vi "Set SplitterPosition.vi"(8 "error in (no error)":errorcluster caption="错误输入（无错误）", 10 "Position(relative)":dbl, 11 "PanelDataNode 输入":refnum<class "PanelDataNode.lvclass"> caption="DNL_LabVIEW Object in") -> (0 "error out":errorcluster caption="错误输出", 3 "PanelDataNode 输出":refnum<class "PanelDataNode.lvclass"> caption="DNL_LabVIEW Object out")   [LabVIEW 2016, in "PanelDataNode.lvclass"]
uses:
  PanelDataNode.lvclass
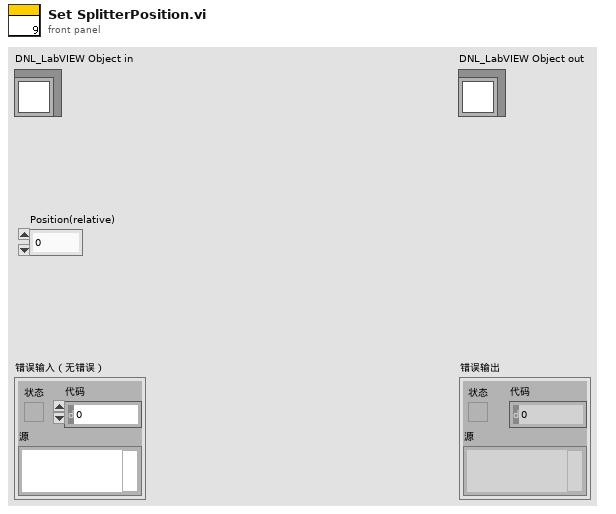
[diagram p1: front panel]
types:
  T1 = typedef "LVBoundsTypeDef.ctl" = cluster{"Width":u32, "Height":u32}
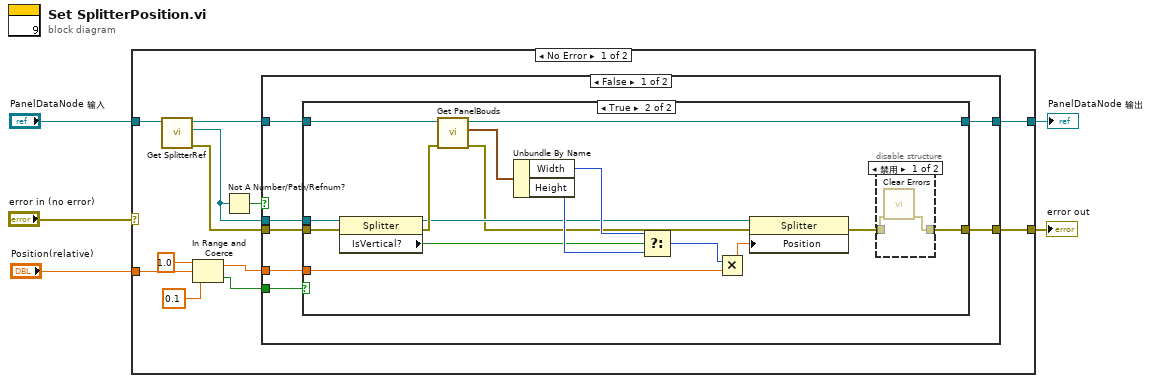
[diagram p0: block diagram]
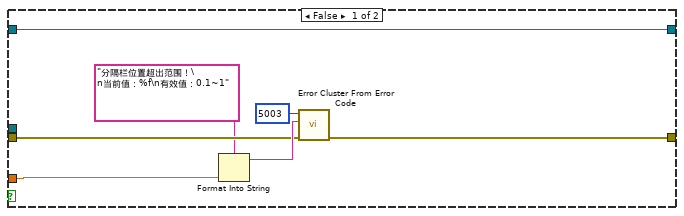
[diagram p2: hidden frame]
diagram:
  n1 = case shown="No Error" "error in (no error)" {
    selector: "error in (no error)" -> [_ w54]
    tunnel: [w13 w54] -> w4
    tunnel: [w14 w53] -> w2
    tunnel: "PanelDataNode 输入" -> [w17 w53]
    tunnel: "Position(relative)" -> [w8 _]
    frame No Error {
      n2 = call "Get SplitterRef.vi"("PanelDataNode 输入"=w17) -> ("error out"=w15:errorcluster, "Splitter"=w11:refnum<vi>, "PanelDataNode 输出"=w16:refnum<class "PanelDataNode.lvclass">)  [unwired: 8 in]
      n3 = In Range and Coerce(upper limit=1.0 ("上限"), x=w8, lower limit=0.1 ("下限")) -> (coerced(x)=w7:dbl, In Range?=w6:bool)
      n4 = Not A Number/Path/Refnum?(number/path/refnum=w11) -> (NaN/Path/Refnum?=w12:bool)
      n5 = case shown="False" w12 {
        tunnel: w16 -> [w24 w52]
        tunnel: w7 -> [w23 _]
        tunnel: w11 -> [w22 _]
        tunnel: w15 -> [w21 w51]
        tunnel: [w20 w52] -> w14
        tunnel: [w19 w51] -> w13
        tunnel: w6 -> [w18 _]
        frame False {
          n6 = case shown="True" w18 {
            tunnel: w24 -> [w25 w47]
            tunnel: w23 -> [w30 w42]
            tunnel: w22 -> [_ w41]
            tunnel: w21 -> [w29 w40]
            tunnel: [w25 w38] -> w20
            tunnel: [w28 w32] -> w19
            frame False {
              n7 = Format Into String(format string="分隔栏位置超出范围！\n当前值：%f\n有效值：0.1~1" ("格式字符串"), w30) -> (resulting string=w31:string)  [unwired: 2 in, 1 out]
              n8 = call <vilib>:"Error Cluster From Error Code.vi"("error in (no error)"=w29, "error message (\"\")"=w31, "error code (0)"=5003) -> ("error out"=w28:errorcluster)  [unwired: 6 in]
            }
            frame True {
              n9 = property class="Splitter"(reference=w41, error in=w40) -> (reference out=w36:refnum<vi>, error out=w39:errorcluster, "IsVertical?"=w37:bool)
              n10 = call "Get PanelBouds.vi"("error in (no error)"=w39, "PanelDataNode 输入"=w47) -> ("error out"=w35:errorcluster, "Bounds"=w44:T1, "PanelDataNode 输出"=w38:refnum<class "PanelDataNode.lvclass">)  [unwired: 7 in]
              n11 = Unbundle By Name(w44) -> ("Width"=w45:u32, "Height"=w46:u32)
              n12 = Select(t=w45, s=w37, f=w46) -> (s? t:f=w43:u32)
              n13 = Multiply(x=w43, y=w42) -> (x*y=w34:dbl)
              n14 = property class="Splitter"(reference=w36, error in=w35, "Position"=w34) -> (error out=w33:errorcluster)  [unwired: 1 out]
              n15 = disable-structure shown="禁用" {
                disable-tunnel: w33 -> [w49 w50]
                disable-tunnel: [w48 w50] -> w32
                frame Disabled {
                  n16 = call <vilib>:"Clear Errors.vi"("error in (no error)"=w49) -> ("error out"=w48:errorcluster)  [unwired: 5 in, 1 out]
                }
                frame Enabled {
                }
              }
            }
          }
        }
        frame True {
        }
      }
    }
    frame Error {
    }
  }
  "error out" <- w4
  "PanelDataNode 输出" <- w2
